vi "DeleteFiles.vi"(6 "delay Command":u32=500, 8 "delay Input":u32=500, 9 "File name string":string="*IDN?\n", 10 "Command String":string="*IDN?\n", 11 "VISA Refnum in":refnum<visa-resource-name>="COM1") -> ()   [LabVIEW 2012]
uses:
  <vilib>/Instr/_visa.llb/VISA Configure Serial Port (Instr).vi
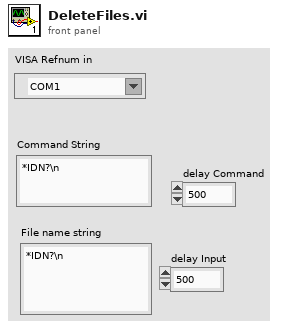
[diagram p1: front panel]
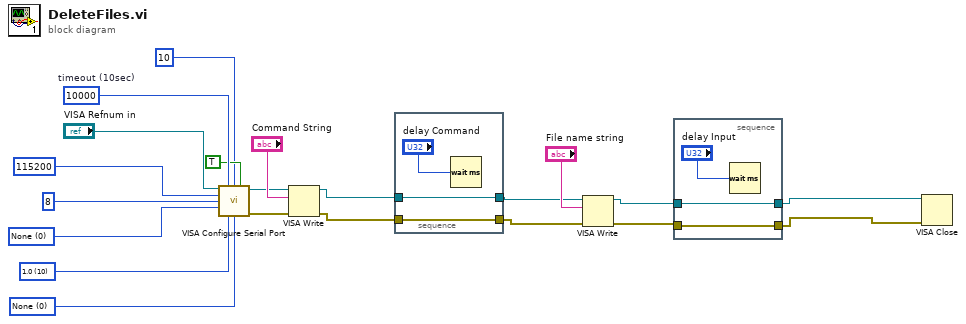
[diagram p0: block diagram]
diagram:
  w21 = u16 0 items=["None"=0, "XON/XOFF"=1, "RTS/CTS"=2, "DTR/DSR"=4] ("flow control")
  w20 = u16 10 items=["1.0"=10, "1.5"=15, "2.0"=20] ("stop bits")
  w19 = u16 0 items=["None", "Odd", "Even", "Mark", "Space"] ("parity")
  w15 = u32 10000  # timeout (10sec)
  n1 = call-poly "VISA Configure Serial Port"("VISA resource name"="VISA Refnum in", "timeout (10sec)"=w15, "termination char\n(0xA = '\\n' = LF)"=u8 10 ("termination char\n(0xA = '\\n' = LF)"), "Enable Termination\nChar (T)"=TRUE ("Enable Termination\nChar (T)"), "baud rate (9600)"=u32 115200 ("baud rate"), "data bits (8)"=u16 8 ("data bits"), "parity (0:none)"=w19, "stop bits (10: 1 bit)"=w20, "flow control (0:none)"=w21) -> ("VISA resource name out"=w13:refnum<visa-resource-name>, "error out"=w12:errorcluster)  [unwired: 1 in, 4 out]
  n2 = VISA Write(VISA resource name=w13, write buffer="Command String", error in (no error)=w12) -> (VISA resource name out=w9:refnum<visa-resource-name>, error out=w8:errorcluster)  [unwired: 1 out]
  n3 = stacked-sequence {
    tunnel: w8 -> [w24]
    tunnel: [w24] -> w5
    tunnel: w9 -> [w23]
    tunnel: [w23] -> w6
    frame #0 {
      n4 = Wait (ms)(milliseconds to wait="delay Command") -> ()  [unwired: 1 out]
    }
  }
  n5 = VISA Write(VISA resource name=w6, write buffer="File name string", error in (no error)=w5) -> (VISA resource name out=w4:refnum<visa-resource-name>, error out=w3:errorcluster)  [unwired: 1 out]
  n6 = stacked-sequence {
    tunnel: w3 -> [w27]
    tunnel: [w27] -> w1
    tunnel: w4 -> [w26]
    tunnel: [w26] -> w2
    frame #0 {
      n7 = Wait (ms)(milliseconds to wait="delay Input") -> ()  [unwired: 1 out]
    }
  }
  n8 = VISA Close(VISA resource name=w2, error in (no error)=w1) -> ()  [unwired: 1 out]
